vi "Update myDouble.vi"(8 "error in (no error)":errorcluster, 10 "myDouble":dbl, 11 "PVClient-Example in":refnum<class "PVClient-Example.lvclass">) -> (0 "error out":errorcluster, 3 "PVClient-Example out":refnum<class "PVClient-Example.lvclass">)   [LabVIEW 2012, in "PVClient-Example.lvlib" / "PVClient-Example.lvclass"]
uses:
  PVClient-Example.lvclass
  PVClient-Example.lvclass/PVClient-Example.ctl
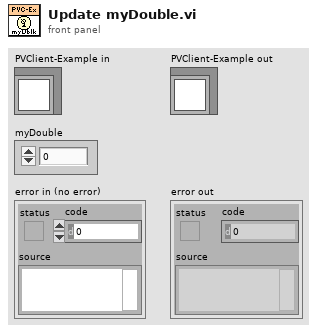
[diagram p1: front panel]
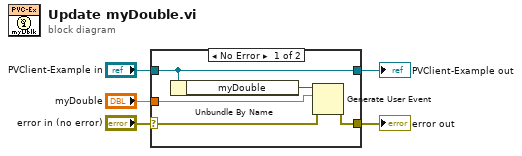
[diagram p0: block diagram]
diagram:
  n1 = case shown="No Error" "error in (no error)" {
    selector: "error in (no error)" -> [w7 w12]
    tunnel: [w6 w12] -> w4
    tunnel: [w10 w11] -> w2
    tunnel: "PVClient-Example in" -> [w10 w11]
    tunnel: "myDouble" -> [w8 _]
    frame No Error {
      n2 = Unbundle By Name(w10) -> ("myDouble"=w9:refnum<user-event>)
      n3 = Generate User Event(user event=w9, event data cluster=w8, error in=w7) -> (error out=w6:errorcluster)  [unwired: 1 out]
    }
    frame Error {
    }
  }
  "error out" <- w4
  "PVClient-Example out" <- w2
